vi "总磷通讯.vi"() -> ()   [LabVIEW 2016, in "总磷.lvlib"]
uses:
  <vilib>/Plasmionique/MB Master/MB_Master_Serial/MB_Master_Serial.lvclass
  C:/PF/National Instruments/LabVIEW 2016/vi.lib/Plasmionique/MB Master/MB_Master/MB_Master.lvclass
  <vilib>/Utility/config.llb/Write Key (Boolean).vi
  <vilib>/Utility/config.llb/Write Key (String).vi
  <vilib>/Utility/config.llb/Read Key (Boolean).vi
  <vilib>/Utility/config.llb/Read Key (String).vi
  <vilib>/Plasmionique/MB Master/MB_Master/MB_Master.lvclass
  <vilib>/Utility/config.llb/NI_LVConfig.lvlib
  <vilib>/Plasmionique/MB Master/MB Master.lvlib
  <vilib>/ptbypt/NI_PtbyPt.lvlib
panel:
  out "序列号":string
  out "状态告警区":T1
  out "测量数据区":T2 {"单位" items=["ug/L", "mg/L", "ppm", "mg/m3", "cm", "ppb", "ug/m3", "%", "nmol/mol", "umol/mol", "MPN/L", "MPN/100ml", "ng/m3", "NTU", "无量纲", "ms/cm", "us/cm", "℃", "mV", "万个/L"]}
  out "status":bool
  out "关键参数区":T3
  in  "读关键参数区":bool
  in  "读状态告警区":bool
  in  "读测量数据区":bool
  in  "站号":u16(ring) items=["总磷"=1, "氨氮"=3]
  in  "停止":bool
  in  "启动":bool
  in  "控制命令":u16(ring) items=["启动测量"=1, "标样核查"=2, "零点核查"=3, "跨度核查"=4, "空白测试"=5, "平行样测试"=6, "加标回收"=7, "空白校准"=8, "标样校准"=9, "初始化（清洗）"=10, "停止测试"=11, "仪器重启"=12, "校时"=13, "模式设置"=14, "测量间隔设置"=15]
  in  "控制命令参数":u16[](array[numeric]) format="%04xH"
  in  "VISA Resource":refnum<visa-resource-name>
  in  "启用模块":bool
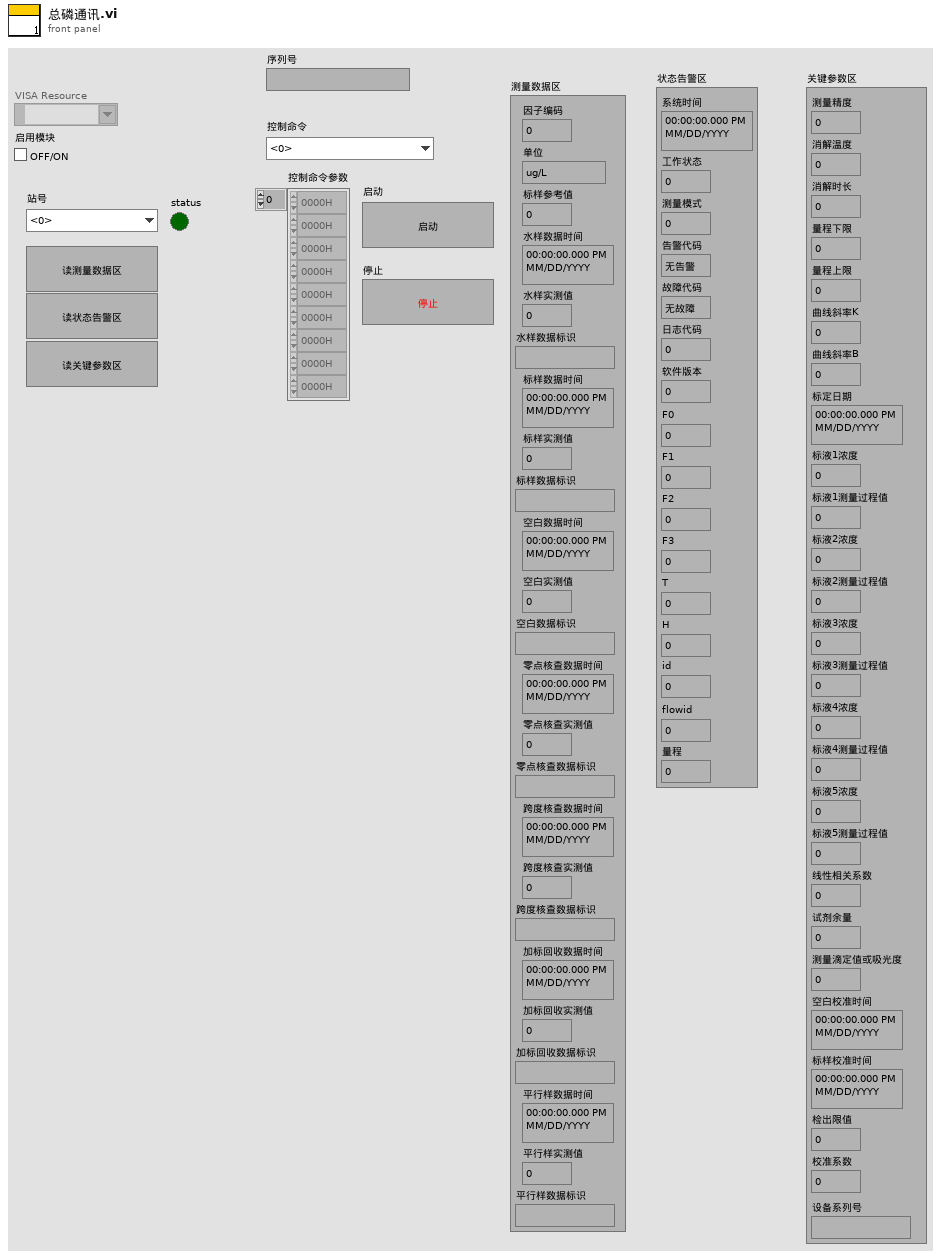
[diagram p1: front panel]
types:
  T1 = cluster{"系统时间":timestamp, "工作状态":u16, "测量模式":u16, "告警代码":enum16{"无告警", "缺试剂告警", "缺水样告警", "缺蒸馏水告警", "缺标液告警", "仪表漏液告警", "标定异常告警", "超量程告警", "加热异常", "低试剂预警", "超上限告警", "超下限告警", "仪表内部其他异常", "滴定异常告警", "电极异常告警", "量程切换告警", "参数设置告警", "PH电极电位异常", "电导率电极异常", "浊度光度异常", "溶解氧电极异常", "溶解氧光强异常", "温度异常告警", "PH异常告警", "溶解氧异常告警", "电导率异常告警", "浊度异常告警", "叶绿素异常告警", "藻密度异常告警", "蓝绿藻异常告警", "ORP异常告警", "氨氮异常告警", "清洁刷异常告警", "SD卡异常告警", "蓝牙异常告警", "Wifi异常告警", "流程异常告警"}, "故障代码":enum16{"无故障", "电机故障", "温度故障", "通讯故障", "滴定故障"}, "日志代码":u16, "软件版本":u16, "F0":sgl, "F1":sgl, "F2":sgl, "F3":sgl, "T":sgl, "H":sgl, "id":u16, "flowid":u16, "量程":u16}
  T2 = cluster{"因子编码":u32, "单位":u16, "标样参考值":sgl, "水样数据时间":timestamp, "水样实测值":sgl, "水样数据标识":string, "标样数据时间":timestamp, "标样实测值":sgl, "标样数据标识":string, "空白数据时间":timestamp, "空白实测值":sgl, "空白数据标识":string, "零点核查数据时间":timestamp, "零点核查实测值":sgl, "零点核查数据标识":string, "跨度核查数据时间":timestamp, "跨度核查实测值":sgl, "跨度核查数据标识":string, "加标回收数据时间":timestamp, "加标回收实测值":sgl, "加标回收数据标识":string, "平行样数据时间":timestamp, "平行样实测值":sgl, "平行样数据标识":string}
  T3 = cluster{"测量精度":u16, "消解温度":u16, "消解时长":u16, "量程下限":sgl, "量程上限":sgl, "曲线斜率K":sgl, "曲线斜率B":sgl, "标定日期":timestamp, "标液1浓度":sgl, "标液1测量过程值":sgl, "标液2浓度":sgl, "标液2测量过程值":sgl, "标液3浓度":sgl, "标液3测量过程值":sgl, "标液4浓度":sgl, "标液4测量过程值":sgl, "标液5浓度":sgl, "标液5测量过程值":sgl, "线性相关系数":sgl, "试剂余量":u32, "测量滴定值或吸光度":sgl, "空白校准时间":timestamp, "标样校准时间":timestamp, "检出限值":sgl, "校准系数":sgl, "设备系列号":string}
  T4 = typedef "NI_LVConfig.lvlib/Config Data RefNum.ctl" = refnum<k1>
  T5 = enum8{"Enabled", "Disabled", "Disabled and Grayed Out"}
  T6 = cluster{"baud rate (bps)":u32, "stop bits":u16, "parity":u16, "flow control":u16, "timeout":u32, "retries":i32}
  T7 = cluster{"系统时间":timestamp, "工作状态":enum16{"空闲", "水样测试", "标样核查", "零点核查", "跨度核查", "空白测试", "平行样测试", "加标回收", "空白校准", "标样校准", "初始化（清洗）"}, "测量模式":enum16{"待机", "连续模式", "周期模式", "定点模式", "受控模式", "手动模式"}, "告警代码":enum16{"无告警", "缺试剂告警", "缺水样告警", "缺蒸馏水告警", "缺标液告警", "仪表漏液告警", "标定异常告警", "超量程告警", "加热异常", "低试剂预警", "超上限告警", "超下限告警", "仪表内部其他异常", "滴定异常告警", "电极异常告警", "量程切换告警", "参数设置告警", "PH电极电位异常", "电导率电极异常", "浊度光度异常", "溶解氧电极异常", "溶解氧光强异常", "温度异常告警", "PH异常告警", "溶解氧异常告警", "电导率异常告警", "浊度异常告警", "叶绿素异常告警", "藻密度异常告警", "蓝绿藻异常告警", "ORP异常告警", "氨氮异常告警", "清洁刷异常告警", "SD卡异常告警", "蓝牙异常告警", "Wifi异常告警", "流程异常告警"}, "故障代码":enum16{"无故障", "电机故障", "温度故障", "通讯故障", "滴定故障"}, "日志代码":u16, "软件版本":u16, "F0":sgl, "F1":sgl, "F2":sgl, "F3":sgl, "T":sgl, "H":sgl, "id":u16, "flowid":u16, "量程":u16}
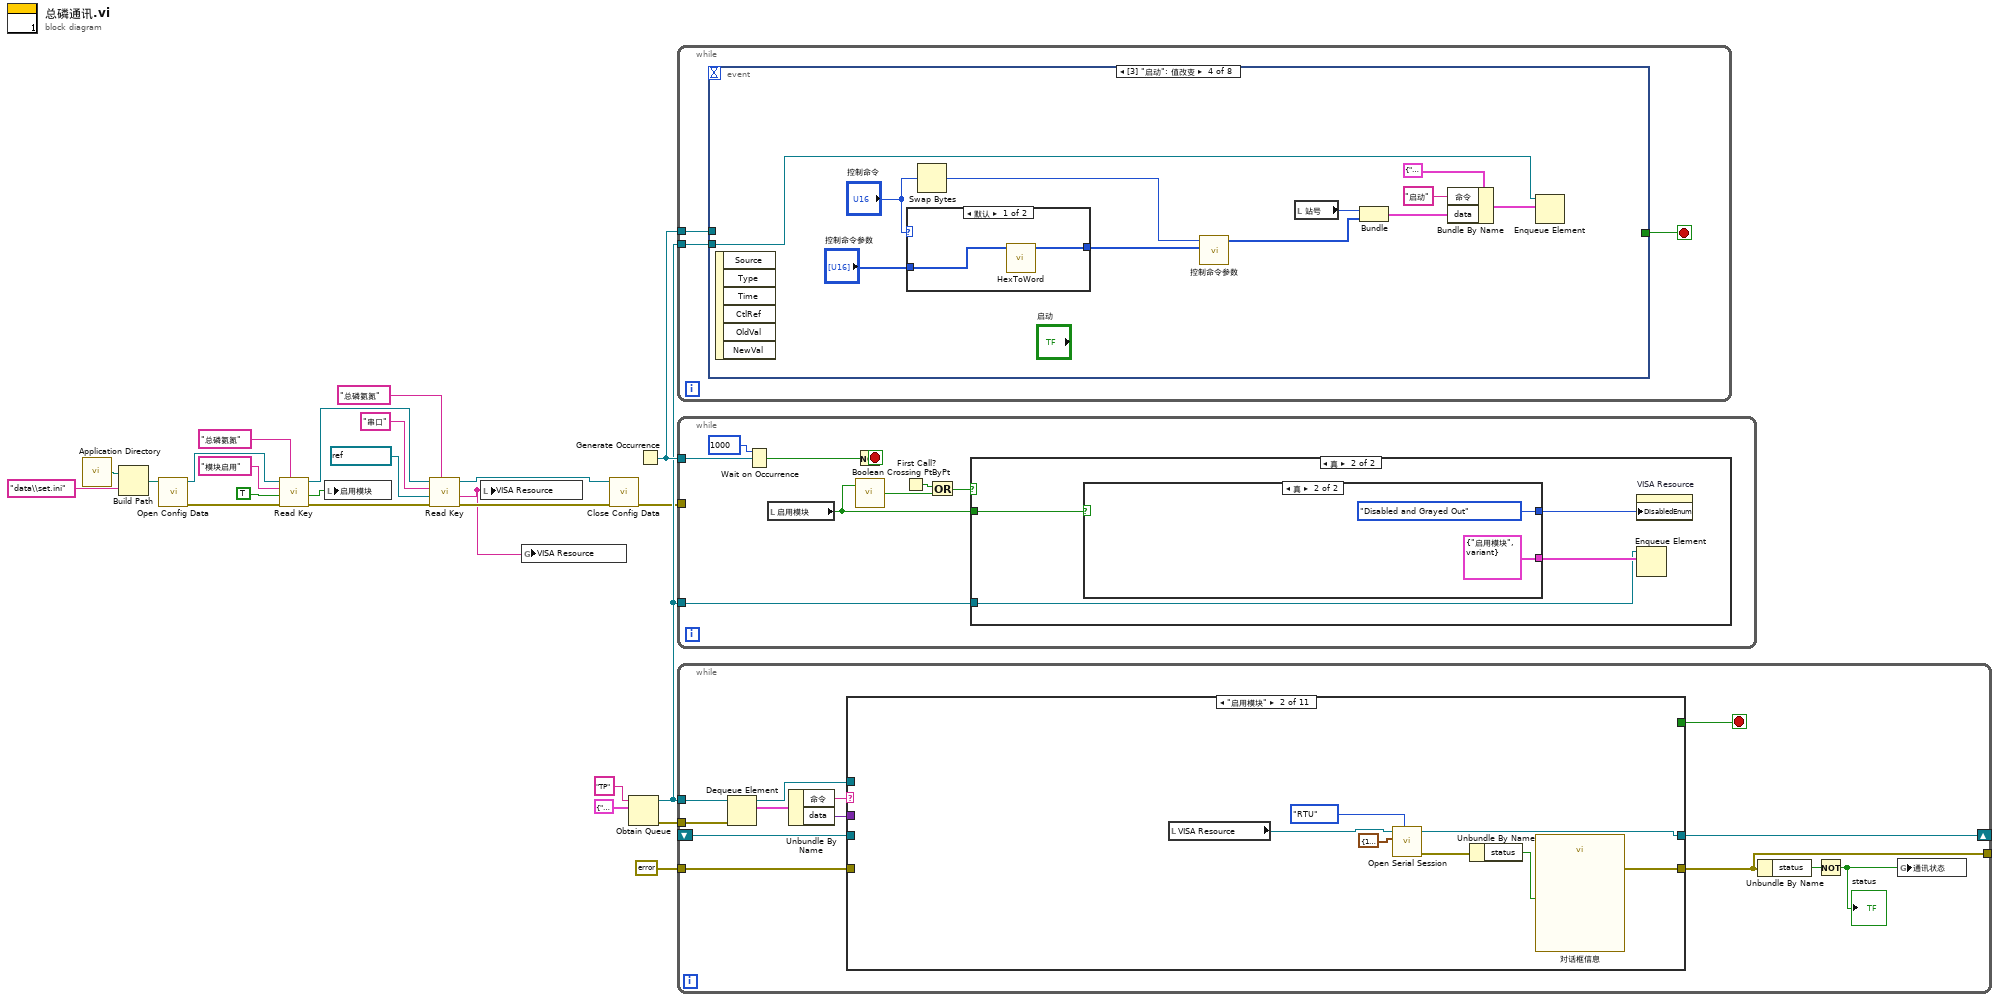
[diagram p0: block diagram]
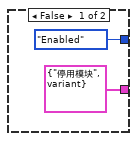
[diagram p3: hidden frame]
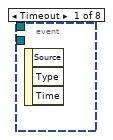
[diagram p4: hidden frame]
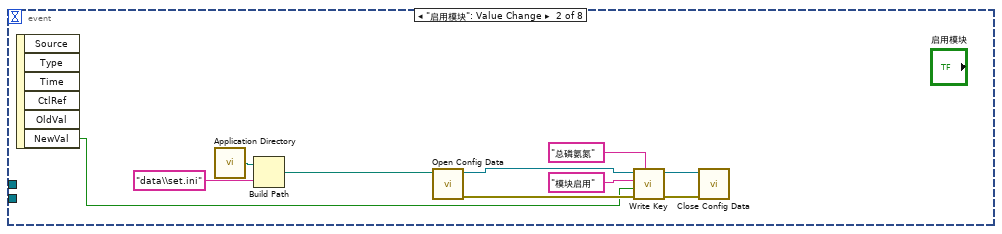
[diagram p5: hidden frame]
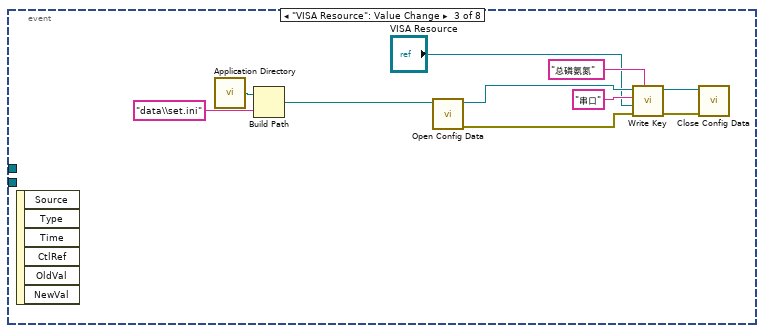
[diagram p6: hidden frame]
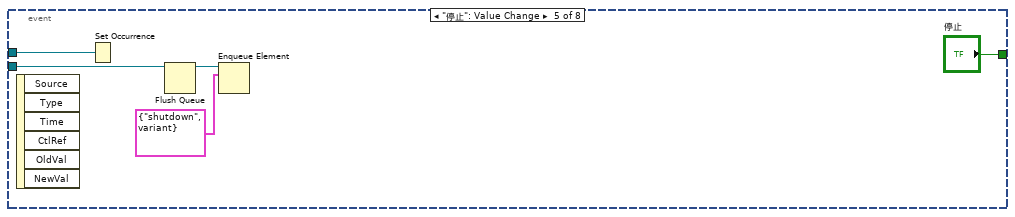
[diagram p8: hidden frame]
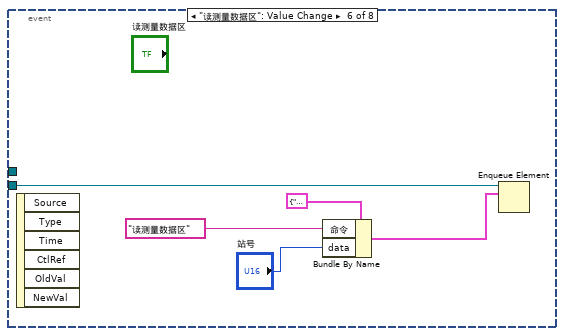
[diagram p9: hidden frame]
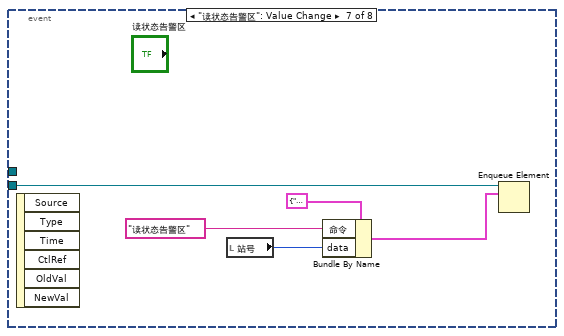
[diagram p10: hidden frame]
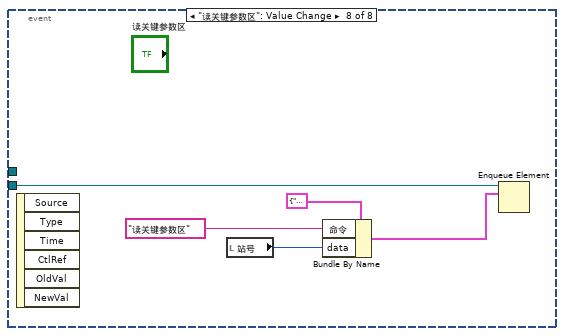
[diagram p11: hidden frame]
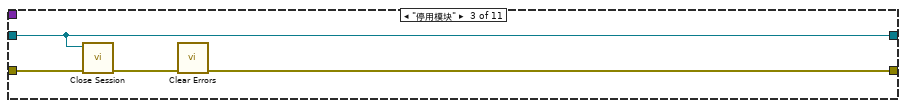
[diagram p13: hidden frame]
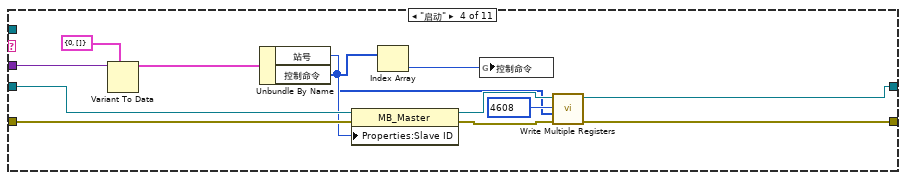
[diagram p14: hidden frame]
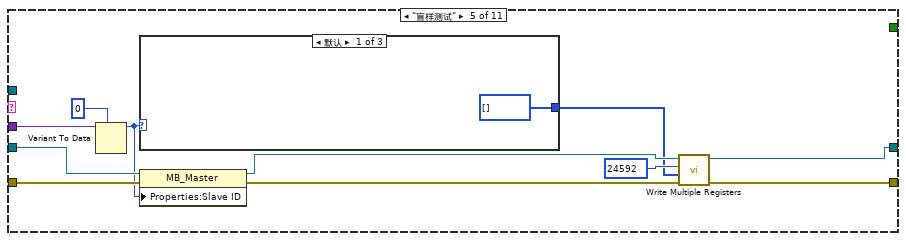
[diagram p15: hidden frame]
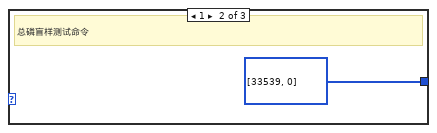
[diagram p16: hidden frame]
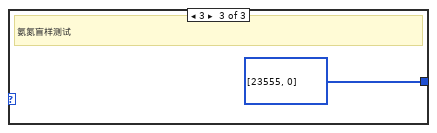
[diagram p17: hidden frame]
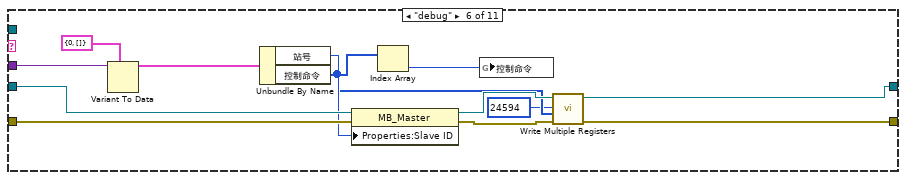
[diagram p18: hidden frame]
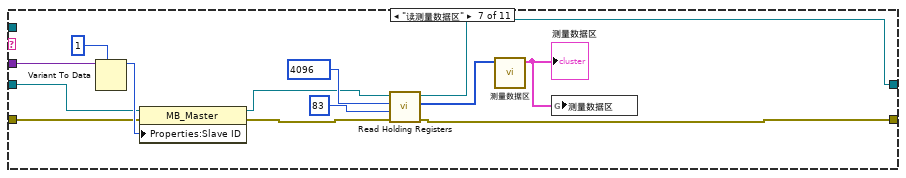
[diagram p19: hidden frame]
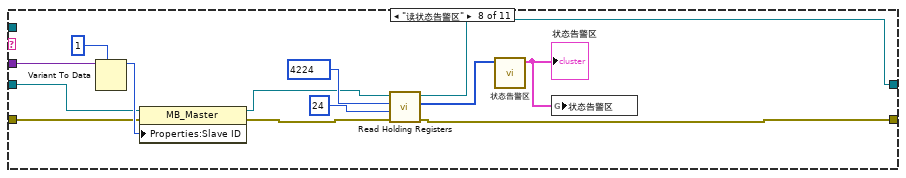
[diagram p20: hidden frame]
diagram:
  n1 = call <vilib>:"Application Directory.vi"() -> ("Application Directory"=w12:path)
  n2 = Build Path(base path=w12, name or relative path="data\\set.ini" ("名称或相对路径")) -> (appended path=w13:path)
  n3 = call <vilib>:"Open Config Data.vi"("configuration file path"=w13) -> ("error out"=w18:errorcluster, "refnum"=w17:T4)  [unwired: 8 in, 1 out]
  n4 = call-poly <vilib>:"Read Key.vi"("section"="总磷氨氮", "error in (no error)"=w18, "default value"=TRUE ("启用模块"), "key"="模块启用", "refnum"=w17) -> ("error out"=w6:errorcluster, "value"=w9:bool, "refnum out"=w8:T4)  [unwired: 3 in, 1 out]
  n5 = local write "启用模块"(w9) -> ()
  n6 = call-poly <vilib>:"Read Key.vi"("section"="总磷氨氮", "error in (no error)"=w6, "default value"=refnum<visa-resource-name> "COM4" ("VISA Resource"), "key"="串口", "refnum"=w8) -> ("error out"=w5:errorcluster, "value"=w1:string, "refnum out"=w7:T4)  [unwired: 3 in, 1 out]
  n7 = local write "VISA Resource"(w1) -> ()
  n8 = global write "VAR总磷氨氮全局变量.vi" "VISA Resource"(w1) -> ()
  n9 = call <vilib>:"Close Config Data.vi"("error in (no error)"=w5, "refnum"=w7) -> ("error out"=w10:errorcluster)  [unwired: 8 in, 1 out]
  n10 = Obtain Queue(name (unnamed)="TP" ("名称（未命名）"), element data type=cluster{"命令":string, "data":variant} {"命令"="", "data"=variant}) -> (queue out=w19:refnum<queue>, error out=w22:errorcluster)  [unwired: 3 in, 1 out]
  n11 = Generate Occurrence() -> (w20:refnum<k4>)
  n12 = while {
    tunnel: w19 -> [w27]
    tunnel: w20 -> [w25]
    stop <- w26 stop-if-true
    n13 = event shown="[3] \"启动\": 值改变" {
      selector: _ -> [_ _ _ _ _ _ _ _]
      dyn-events: _ -> [_ _ _ _ _ _ _ _]
      timeout: _ -> [_ _ _ _ _ _ _ _]
      tunnel: w27 -> [_ _ _ w58 w65 w71 w76 w81]
      tunnel: [_ _ _ _ "停止" _ _ _] -> w26
      tunnel: w25 -> [_ _ _ _ w62 _ _ _]
      event Timeout {
        n14 = event-data() -> ()  [unwired: 1 in, 3 out]
      }
      event "启用模块": Value Change {
        n15 = event-data() -> ("NewVal"=w28:bool)  [unwired: 1 in, 5 out]
        n16 = call <vilib>:"Application Directory.vi"() -> ("Application Directory"=w30:path)
        n17 = Build Path(base path=w30, name or relative path="data\\set.ini" ("名称或相对路径")) -> (appended path=w31:path)
        n18 = call <vilib>:"Open Config Data.vi"("configuration file path"=w31) -> ("error out"=w37:errorcluster, "refnum"=w36:T4)  [unwired: 8 in, 1 out]
        n19 = call-poly <vilib>:"Write Key.vi"("section"="总磷氨氮", "error in (no error)"=w37, "value"=w28, "key"="模块启用", "refnum"=w36) -> ("error out"=w33:errorcluster, "refnum out"=w29:T4)  [unwired: 4 in, 1 out]
        n20 = call <vilib>:"Close Config Data.vi"("error in (no error)"=w33, "refnum"=w29) -> ()  [unwired: 8 in, 2 out]
      }
      event "VISA Resource": Value Change {
        n21 = event-data() -> ()  [unwired: 1 in, 6 out]
        n22 = call <vilib>:"Application Directory.vi"() -> ("Application Directory"=w40:path)
        n23 = Build Path(base path=w40, name or relative path="data\\set.ini" ("名称或相对路径")) -> (appended path=w41:path)
        n24 = call <vilib>:"Open Config Data.vi"("configuration file path"=w41) -> ("error out"=w47:errorcluster, "refnum"=w46:T4)  [unwired: 8 in, 1 out]
        n25 = call-poly <vilib>:"Write Key.vi"("section"="总磷氨氮", "error in (no error)"=w47, "value"="VISA Resource", "key"="串口", "refnum"=w46) -> ("error out"=w43:errorcluster, "refnum out"=w39:T4)  [unwired: 4 in, 1 out]
        n26 = call <vilib>:"Close Config Data.vi"("error in (no error)"=w43, "refnum"=w39) -> ()  [unwired: 8 in, 2 out]
      }
      event "启动": Value Change {
        n27 = event-data() -> ()  [unwired: 1 in, 6 out]
        n28 = case shown="默认" "控制命令" {
          tunnel: "控制命令参数" -> [w60 w61]
          tunnel: [w59 w61] -> w48
          frame Default {
            n29 = call "HexToWord.vi"("数组"=w60) -> ("WORD"=w59:u16[])  [unwired: 10 in]
          }
          frame 13 {
          }
        }
        n30 = Swap Bytes(anything="控制命令") -> (byte swapped=w51:u16)
        n31 = call "控制命令参数.vi"("控制命令参数"=w48, "控制命令"=w51) -> ("控制命令输出"=w54:u16[])  [unwired: 9 in]
        n32 = local read "站号"() -> (w53:u16)
        n33 = Bundle("站号"=w53, "控制命令输出"=w54) -> (w52:cluster{"站号":u16, "控制命令输出":u16[]})  [unwired: 1 in]
        n34 = Bundle By Name(cluster=cluster{"命令":string, "data":variant} {"命令"="", "data"=variant} ("元素"), "命令"="启动", "data"=w52) -> (w56:cluster{"命令":string, "data":variant})
        n35 = Enqueue Element(queue=w58, element=w56) -> ()  [unwired: 2 in, 3 out]
      }
      event "停止": Value Change {
        n36 = event-data() -> ()  [unwired: 1 in, 6 out]
        n37 = Set Occurrence(w62) -> ()
        n38 = Flush Queue(queue=w65) -> (queue out=w64:refnum<queue>)  [unwired: 1 in, 2 out]
        n39 = Enqueue Element(queue=w64, element=cluster{"命令":string, "data":variant} {"命令"="shutdown", "data"=variant} ("元素")) -> ()  [unwired: 2 in, 3 out]
      }
      event "读测量数据区": Value Change {
        n40 = event-data() -> ()  [unwired: 1 in, 6 out]
        n41 = Bundle By Name(cluster=cluster{"命令":string, "data":variant} {"命令"="", "data"=variant} ("元素"), "命令"="读测量数据区", "data"="站号") -> (w69:cluster{"命令":string, "data":variant})
        n42 = Enqueue Element(queue=w71, element=w69) -> ()  [unwired: 2 in, 3 out]
      }
      event "读状态告警区": Value Change {
        n43 = event-data() -> ()  [unwired: 1 in, 6 out]
        n44 = local read "站号"() -> (w72:u16)
        n45 = Bundle By Name(cluster=cluster{"命令":string, "data":variant} {"命令"="", "data"=variant} ("元素"), "命令"="读状态告警区", "data"=w72) -> (w74:cluster{"命令":string, "data":variant})
        n46 = Enqueue Element(queue=w76, element=w74) -> ()  [unwired: 2 in, 3 out]
      }
      event "读关键参数区": Value Change {
        n47 = event-data() -> ()  [unwired: 1 in, 6 out]
        n48 = local read "站号"() -> (w77:u16)
        n49 = Bundle By Name(cluster=cluster{"命令":string, "data":variant} {"命令"="", "data"=variant} ("元素"), "命令"="读关键参数区", "data"=w77) -> (w79:cluster{"命令":string, "data":variant})
        n50 = Enqueue Element(queue=w81, element=w79) -> ()  [unwired: 2 in, 3 out]
      }
    }
  }
  n51 = while {
    tunnel: w20 -> [w90]
    tunnel: w19 -> [w85]
    tunnel: w10 -> [_]
    stop <- w87 stop-if-true
    n52 = Wait on Occurrence(2:w90, 3:1000 ("毫秒超时(-1)")) -> (0:w88:bool)  [unwired: 1 in]
    n53 = local read "启用模块"() -> (w86:bool)
    n54 = Not(x=w88) -> (.not. x?=w87:bool)
    n55 = call <vilib>:"Boolean Crossing PtByPt.vi"("input"=w86) -> ("crossing"=w83:bool)  [unwired: 2 in]
    n56 = First Call?() -> (First Call?: T/F=w84:bool)
    n57 = Or(x=w84, y=w83) -> (x .or. y?=w82:bool)
    n58 = case shown="真" w82 {
      tunnel: w86 -> [_ w93]
      tunnel: w85 -> [_ w92]
      frame False {
      }
      frame True {
        n59 = case shown="真" w93 {
          tunnel: [cluster{"命令":string, "data":variant} {"命令"="停用模块", "data"=variant} ("元素") cluster{"命令":string, "data":variant} {"命令"="启用模块", "data"=variant} ("元素")] -> w94
          tunnel: [T5."Enabled" ("禁用") T5."Disabled and Grayed Out" ("禁用")] -> w91
          frame False {
          }
          frame True {
          }
        }
        n60 = property on="VISA Resource" class="VISAName"("DisabledEnum"=w91) -> ()  [unwired: 2 in, 2 out]
        n61 = Enqueue Element(queue=w92, element=w94) -> ()  [unwired: 2 in, 3 out]
      }
    }
  }
  n62 = while {
    tunnel: w19 -> [w111]
    tunnel: w22 -> [w110]
    shift-right: [w108] -> _
    shift-left: _ -> [w107]
    tunnel: errorcluster {"status"=FALSE, "code"=0, "source"=""} ("error out") -> [w106]
    tunnel: [w101] -> _
    stop <- w109 stop-if-true
    n63 = Dequeue Element(queue=w111, error in (no error)=w110) -> (queue out=w102:refnum<queue>, element=w104:cluster{"命令":string, "data":variant})  [unwired: 1 in, 2 out]
    n64 = Unbundle By Name(w104) -> ("命令"=w105:string, "data"=w103:variant)
    n65 = case shown="\"启用模块\"" w105 {
      tunnel: w103 -> [_ _ _ w134 w145 w162 w171 w180 w195 w209 _]
      tunnel: w102 -> [_ _ _ _ _ _ _ _ _ _ w222]
      tunnel: [_ _ _ _ _ _ _ _ _ _ TRUE] -> w109
      tunnel: [w112 w120 w121 w137 w148 w164 w176 w189 w202 w216 w218] -> w108
      tunnel: [w113 w115 w122 w136 w147 w163 w177 w190 w203 w217 w219] -> w101
      tunnel: w107 -> [w112 _ w121 w133 w144 w161 w170 w183 w198 w212 w218]
      tunnel: w106 -> [w113 _ w124 w130 w141 w158 w168 w184 w199 w213 w220]
      frame Default {
      }
      frame "启用模块" {
        n66 = local read "VISA Resource"() -> (w114:refnum<visa-resource-name>)
        n67 = call <vilib>:"Open Serial Session.vi"("Mode (RTU)"=enum16{"RTU", "ASCII"}."RTU", "Serial Config"=T6 {"baud rate (bps)"=115200, "stop bits"=10, "parity"=0, "flow control"=0, "timeout"=1000, "retries"=1}, "VISA Resource"=w114) -> ("Error out"=w116:errorcluster, "MB_Serial session"=w120:refnum<class "MB_Master_Serial.lvclass">)  [unwired: 7 in]
        n68 = Unbundle By Name(w116) -> ("status"=w117:bool)
        n69 = call "对话框信息"("Enable"=w117) -> ("error out"=w115:errorcluster)  [unwired: 9 in, 1 out]
      }
      frame "停用模块" {
        n70 = call-dynamic "Close Session.vi"("error in (no error)"=w124, "MB session in"=w121) -> ("error out"=w123:errorcluster)  [unwired: 9 in]
        n71 = call <vilib>:"Clear Errors.vi"("error in (no error)"=w123) -> ("error out"=w122:errorcluster)  [unwired: 5 in, 1 out]
      }
      frame "启动" {
        n72 = Variant To Data(type=cluster{"站号":u16, "控制命令":u16[]} {"站号"=0, "控制命令"=[]} ("输出簇"), Variant=w134) -> (data=w128:cluster{"站号":u16, "控制命令":u16[]})  [unwired: 1 in, 1 out]
        n73 = Unbundle By Name(w128) -> ("站号"=w127:u16, "控制命令"=w125:u16[])
        n74 = property class="MB_Master"(reference=w133, error in=w130, "Properties:Slave ID"=w127) -> (reference out=w132:refnum<class "MB_Master.lvclass">, error out=w131:errorcluster)
        n75 = Index Array(array=w125) -> (element=w126:u16)  [unwired: 1 in]
        n76 = global write "VAR总磷氨氮全局变量.vi" "控制命令"(w126) -> ()
        n77 = call <vilib>:"Write Multiple Registers.vi"("error in (no error)"=w131, "values"=w125, "starting address"=u16 4608, "MB session in"=w132) -> ("error out"=w136:errorcluster, "MB session out"=w137:refnum<class "MB_Master.lvclass">)  [unwired: 6 in]
      }
      frame "盲样测试" {
        n78 = Variant To Data(type=0, Variant=w145) -> (data=w138:i32)  [unwired: 1 in, 1 out]
        n79 = case shown="默认" w138 {
          tunnel: [u16[] [] ("values") u16[] [33539, 0] ("values") u16[] [23555, 0] ("values")] -> w140
          frame Default {
          }
          frame 1 {
            # "总磷盲样测试命令"
          }
          frame 3 {
            # "氨氮盲样测试"
          }
        }
        n80 = property class="MB_Master"(reference=w144, error in=w141, "Properties:Slave ID"=w138) -> (reference out=w143:refnum<class "MB_Master.lvclass">, error out=w142:errorcluster)
        n81 = call <vilib>:"Write Multiple Registers.vi"("error in (no error)"=w142, "values"=w140, "starting address"=u16 24592, "MB session in"=w143) -> ("error out"=w147:errorcluster, "MB session out"=w148:refnum<class "MB_Master.lvclass">)  [unwired: 6 in]
      }
      frame "debug" {
        n82 = Variant To Data(type=cluster{"站号":u16, "控制命令":u16[]} {"站号"=0, "控制命令"=[]} ("输出簇"), Variant=w162) -> (data=w156:cluster{"站号":u16, "控制命令":u16[]})  [unwired: 1 in, 1 out]
        n83 = Unbundle By Name(w156) -> ("站号"=w155:u16, "控制命令"=w153:u16[])
        n84 = property class="MB_Master"(reference=w161, error in=w158, "Properties:Slave ID"=w155) -> (reference out=w160:refnum<class "MB_Master.lvclass">, error out=w159:errorcluster)
        n85 = Index Array(array=w153) -> (element=w154:u16)  [unwired: 1 in]
        n86 = global write "VAR总磷氨氮全局变量.vi" "控制命令"(w154) -> ()
        n87 = call <vilib>:"Write Multiple Registers.vi"("error in (no error)"=w159, "values"=w153, "starting address"=u16 24594, "MB session in"=w160) -> ("error out"=w163:errorcluster, "MB session out"=w164:refnum<class "MB_Master.lvclass">)  [unwired: 6 in]
      }
      frame "读测量数据区" {
        n88 = Variant To Data(type=u8 1 ("Slave ID"), Variant=w171) -> (data=w172:u8)  [unwired: 1 in, 1 out]
        n89 = property class="MB_Master"(reference=w170, error in=w168, "Properties:Slave ID"=w172) -> (reference out=w169:refnum<class "MB_Master.lvclass">, error out=w167:errorcluster)
        n90 = call <vilib>:"Read Holding Registers.vi"("error in (no error)"=w167, "quantity"=u16 83, "starting address"=u16 4096, "MB session in"=w169) -> ("error out"=w177:errorcluster, "Registers"=w166:u16[], "MB session out"=w176:refnum<class "MB_Master.lvclass">)  [unwired: 5 in]
        n91 = call "测量数据区.vi"("数组"=w166) -> ("测量数据区"=w165:T2)  [unwired: 10 in]
        "测量数据区" <- w165
        n92 = global write "VAR总磷氨氮全局变量.vi" "测量数据区"(w165) -> ()
      }
      frame "读状态告警区" {
        n93 = Variant To Data(type=u8 1 ("Slave ID"), Variant=w180) -> (data=w185:u8)  [unwired: 1 in, 1 out]
        n94 = property class="MB_Master"(reference=w183, error in=w184, "Properties:Slave ID"=w185) -> (reference out=w182:refnum<class "MB_Master.lvclass">, error out=w181:errorcluster)
        n95 = call <vilib>:"Read Holding Registers.vi"("error in (no error)"=w181, "quantity"=u16 24, "starting address"=u16 4224, "MB session in"=w182) -> ("error out"=w190:errorcluster, "Registers"=w179:u16[], "MB session out"=w189:refnum<class "MB_Master.lvclass">)  [unwired: 5 in]
        n96 = call "状态告警区.vi"("数组"=w179) -> ("状态告警区"=w178:T7)  [unwired: 10 in]
        "状态告警区" <- w178
        n97 = global write "VAR总磷氨氮全局变量.vi" "状态告警区"(w178) -> ()
      }
      frame "读关键参数区" {
        n98 = Variant To Data(type=u8 1 ("Slave ID"), Variant=w195) -> (data=w193:u8)  [unwired: 1 in, 1 out]
        n99 = property class="MB_Master"(reference=w198, error in=w199, "Properties:Slave ID"=w193) -> (reference out=w197:refnum<class "MB_Master.lvclass">, error out=w196:errorcluster)
        n100 = call <vilib>:"Read Holding Registers.vi"("error in (no error)"=w196, "quantity"=u16 19, "starting address"=u16 4256, "MB session in"=w197) -> ("error out"=w203:errorcluster, "Registers"=w192:u16[], "MB session out"=w202:refnum<class "MB_Master.lvclass">)  [unwired: 5 in]
        n101 = call "关键参数区.vi"("数组"=w192) -> ("关键参数区"=w191:T3)  [unwired: 10 in]
        "关键参数区" <- w191
        n102 = global write "VAR总磷氨氮全局变量.vi" "关键参数区"(w191) -> ()
      }
      frame "读序列号" {
        n103 = Variant To Data(type=u8 1 ("Slave ID"), Variant=w209) -> (data=w207:u8)  [unwired: 1 in, 1 out]
        n104 = property class="MB_Master"(reference=w212, error in=w213, "Properties:Slave ID"=w207) -> (reference out=w211:refnum<class "MB_Master.lvclass">, error out=w210:errorcluster)
        n105 = call <vilib>:"Read Holding Registers.vi"("error in (no error)"=w210, "quantity"=u16 6, "starting address"=u16 3, "MB session in"=w211) -> ("error out"=w217:errorcluster, "Registers"=w206:u16[], "MB session out"=w216:refnum<class "MB_Master.lvclass">)  [unwired: 5 in]
        n106 = call "HexToString.vi"("数组"=w206) -> ("STRING"=w205:string[])  [unwired: 10 in]
        n107 = Index Array(array=w205) -> (element=w204:string)  [unwired: 1 in]
        "序列号" <- w204
        n108 = global write "VAR总磷氨氮全局变量.vi" "序列号"(w204) -> ()
      }
      frame "shutdown" {
        n109 = call-dynamic "Close Session.vi"("error in (no error)"=w220, "MB session in"=w218) -> ("error out"=w219:errorcluster)  [unwired: 9 in]
        n110 = Flush Queue(queue=w222) -> (queue out=w221:refnum<queue>)  [unwired: 1 in, 2 out]
        n111 = Release Queue(queue=w221) -> ()  [unwired: 2 in, 3 out]
      }
    }
    n112 = Unbundle By Name(w101) -> ("status"=w100:bool)
    n113 = Not(x=w100) -> (.not. x?=w99:bool)
    "status" <- w99
    n114 = global write "VAR总磷氨氮全局变量.vi" "通讯状态"(w99) -> ()
  }
